vi "Make Project Path.vi"(11 "Data Cluster":T1) -> (2 "project path":path, 3 "project folder":path)   [LabVIEW 2013, in "Project Wizard.lvlib"]
uses:
  Project Wizard.lvlib
  controls/UI Data.ctl
  controls/Template.ctl
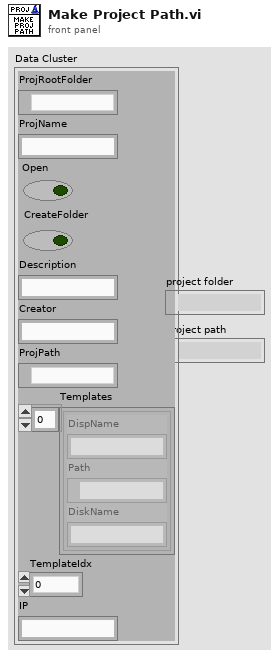
[diagram p1: front panel]
types:
  T1 = typedef "Project Wizard.lvlib/UI Data.ctl" = cluster{"ProjRootFolder":path, "ProjName":string, "Open":bool, "CreateFolder":bool, "Description":string, "Creator":string, "ProjPath":path, "Templates":T2[], "TemplateIdx":u16, "IP":string}
  T2 = typedef "Project Wizard.lvlib/Template.ctl" = cluster{"DispName":string, "Path":path, "DiskName":string}
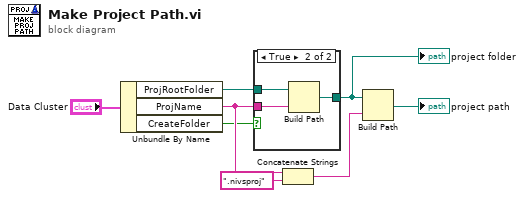
[diagram p0: block diagram]
diagram:
  n1 = Unbundle By Name("Data Cluster") -> ("ProjRootFolder"=w4:path, "ProjName"=w5:string, "CreateFolder"=w3:bool)
  n2 = case shown="True" w3 {
    tunnel: w4 -> [w9 w12]
    tunnel: w5 -> [_ w11]
    tunnel: [w9 w10] -> w1
    frame False {
    }
    frame True {
      n3 = Build Path(base path=w12, name or relative path=w11) -> (appended path=w10:path)
    }
  }
  "project folder" <- w1
  n4 = Concatenate Strings(w5, ".nivsproj" ("string")) -> (w7:string)
  n5 = Build Path(base path=w1, name or relative path=w7) -> (appended path=→"project path":path)
